vi "PC_save_unique_file_certain_time.vi"(6 "Save?":bool, 7 "Waveform":waveform(dbl), 8 "error in (no error)":errorcluster, 9 "Seconds In File":dbl, 11 "File Parameters":T1) -> (0 "error out":errorcluster, 3 "file path out":path)   [LabVIEW 2020]
uses:
  <vilib>/Waveform/WDTOps.llb/WDT Waveform Duration DBL.vi
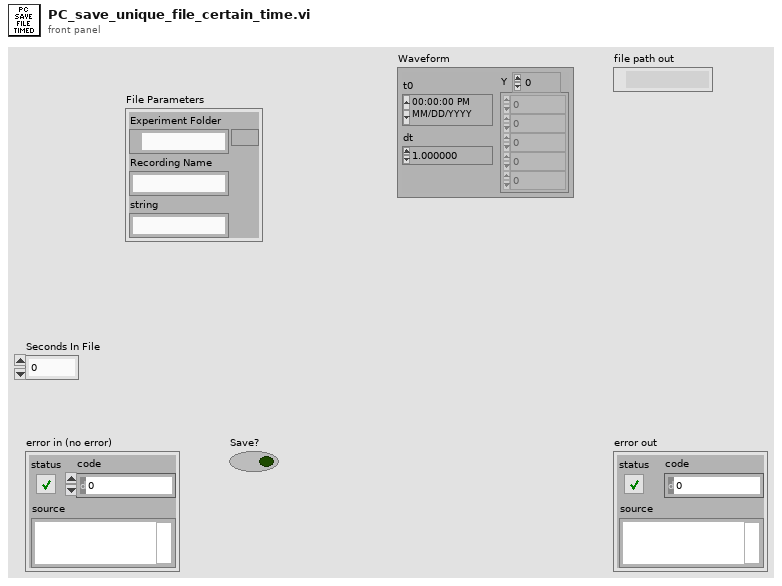
[diagram p1: front panel]
types:
  T1 = cluster{"Experiment Folder":path, "Recording Name":string, "string":string}
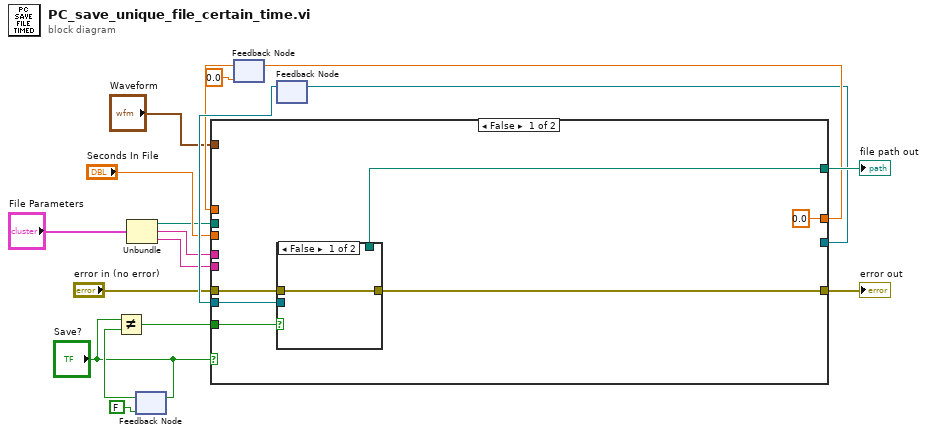
[diagram p0: block diagram]
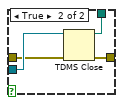
[diagram p2: hidden frame]
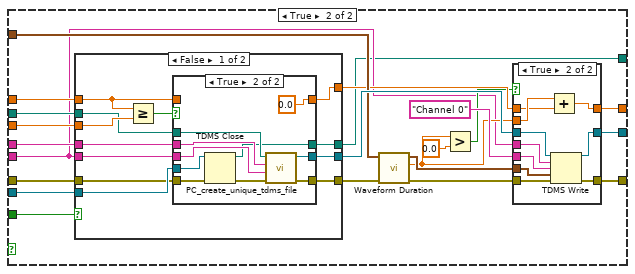
[diagram p3: hidden frame]
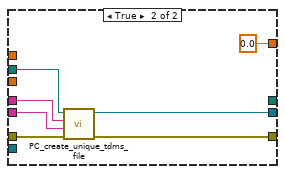
[diagram p6: hidden frame]
diagram:
  n1 = Unbundle("File Parameters") -> ("Experiment Folder"=w4:path, "Recording Name"=w3:string, "string"=w2:string)
  n2 = feedback #1(FALSE ("Save?")) -> (w7:bool)
  n3 = Not Equal?(x="Save?", y=w7) -> (x != y?=w5:bool)
  n4 = feedback-in #1("Save?") -> ()
  n5 = feedback #2(0.0 ("duration")) -> (w14:dbl)
  n6 = feedback #3() -> (w16:refnum<k34>)  [unwired: 1 in]
  n7 = case shown="False" "Save?" {
    tunnel: w5 -> [w23 w51]
    tunnel: w4 -> [_ w50]
    tunnel: w3 -> [_ w49]
    tunnel: w2 -> [_ w32]
    tunnel: "Waveform" -> [_ w45]
    tunnel: "error in (no error)" -> [w21 w47]
    tunnel: [_ w46] -> w11
    tunnel: [0.0 w41] -> w12
    tunnel: w14 -> [_ w40]
    tunnel: "Seconds In File" -> [_ w39]
    tunnel: w16 -> [w22 w38]
    tunnel: [w20 w31] -> w17
    tunnel: [w19 w30] -> w18
    frame False {
      n8 = case shown="False" w23 {
        tunnel: w22 -> [_ w29]
        tunnel: w21 -> [w25 w28]
        tunnel: [w25 w27] -> w20
        tunnel: [_ w26] -> w19
        frame False {
        }
        frame True {
          n9 = TDMS Close(8:w28, 11:w29) -> (0:w27:errorcluster, 3:w26:path)
        }
      }
    }
    frame True {
      n10 = case shown="False" w51 {
        tunnel: w50 -> [w71 w96]
        tunnel: w49 -> [w72 w95]
        tunnel: w32 -> [w73 w94]
        tunnel: [w70 w93] -> w48
        tunnel: [w69 w92] -> w44
        tunnel: w47 -> [w68 w91]
        tunnel: w40 -> [w67 _]
        tunnel: w39 -> [w76 _]
        tunnel: w38 -> [w74 _]
        tunnel: [w66 0.0 ("duration")] -> w37
        tunnel: [w65 _] -> w30
        frame False {
          n11 = Greater Or Equal?(x=w67, y=w76) -> (x >= y?=w75:bool)
          n12 = case shown="True" w75 {
            tunnel: w74 -> [w79 w89]
            tunnel: w73 -> [_ w88]
            tunnel: w72 -> [_ w87]
            tunnel: w71 -> [_ w86]
            tunnel: [w79 w85] -> w70
            tunnel: [w78 w83] -> w69
            tunnel: w68 -> [w78 w82]
            tunnel: w67 -> [w77 _]
            tunnel: [w77 0.0 ("duration")] -> w66
            tunnel: [_ w80] -> w65
            frame False {
            }
            frame True {
              n13 = TDMS Close(8:w82, 11:w89) -> (0:w84:errorcluster, 3:w80:path)
              n14 = call "PC_create_unique_tdms_file.vi"("error in (no error)"=w84, "string"=w88, "Recording Name"=w87, "Experiment Folder"=w86) -> ("error out"=w83:errorcluster, "Refnum out"=w85:refnum<k34>)  [unwired: 6 in]
            }
          }
        }
        frame True {
          n15 = call "PC_create_unique_tdms_file.vi"("error in (no error)"=w91, "string"=w94, "Recording Name"=w95, "Experiment Folder"=w96) -> ("error out"=w92:errorcluster, "Refnum out"=w93:refnum<k34>)  [unwired: 6 in]
        }
      }
      n16 = call-poly <vilib>:"Waveform Duration.vi"("error in (no error)"=w44, "waveform in"=w45) -> ("error out"=w43:errorcluster, "duration"=w35:dbl, "waveform out"=w42:waveform(dbl))  [unwired: 7 in]
      n17 = Greater?(x=w35, y=0.0) -> (0:w33:bool)
      n18 = case shown="True" w33 {
        tunnel: w48 -> [w54 w64]
        tunnel: [w54 w63] -> w46
        tunnel: w43 -> [w52 w62]
        tunnel: w42 -> [_ w61]
        tunnel: w35 -> [_ w60]
        tunnel: [w53 w59] -> w41
        tunnel: w37 -> [w53 w58]
        tunnel: "Channel 0" ("channel name(s) in (Untitled)") -> [_ w57]
        tunnel: w32 -> [_ w56]
        tunnel: [w52 w55] -> w31
        frame False {
        }
        frame True {
          n19 = Add(x=w60, y=w58) -> (x+y=w59:dbl)
          n20 = TDMS Write(0:w64, 5:w56, 7:w57, 9:w61, 11:w62) -> (4:w63:refnum<k34>, 15:w55:errorcluster)  [unwired: 1 in, 2 out]
        }
      }
    }
  }
  "file path out" <- w18
  "error out" <- w17
  n21 = feedback-in #2(w12) -> ()
  n22 = feedback-in #3(w11) -> ()
